vi "ReadMbDat.vi"(0 "ModbusSp in":refnum<class "ModbusSp.lvclass">, 11 "error in (no error)":errorcluster) -> (4 "ModbusSp out":refnum<class "ModbusSp.lvclass">, 6 "Data Read":T1, 8 "register readed":u16[](array[numeric]), 15 "error out":errorcluster)   [LabVIEW 2019, in "ModbusSp.lvclass"]
uses:
  ModbusSp.lvclass
  ReadData.ctl
  ModbusSp.lvclass/ModbusSp.ctl
  Modbus Data Type Conversation/U16 Array TO SGL Array.vi
  <vilib>/NI/Modbus Library/API/Slave/Modbus Slave.lvclass
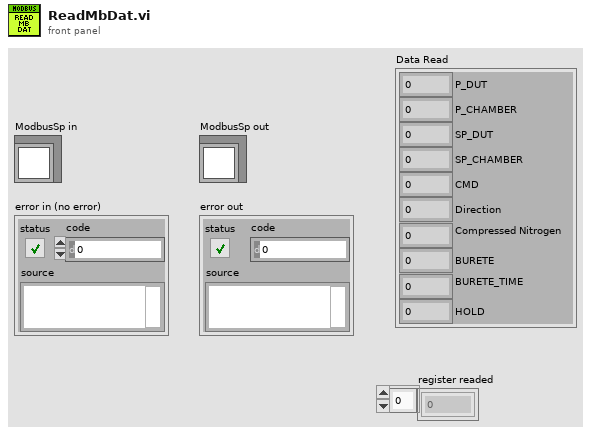
[diagram p1: front panel]
types:
  T1 = typedef "ModbusSp.lvclass/ReadData.ctl" = cluster{"P_DUT":sgl, "P_CHAMBER":sgl, "SP_DUT":sgl, "SP_CHAMBER":sgl, "CMD":u16, "Direction":u16, "Compressed Nitrogen":u16, "BURETE":u16, "BURETE_TIME":u16, "HOLD":u16}
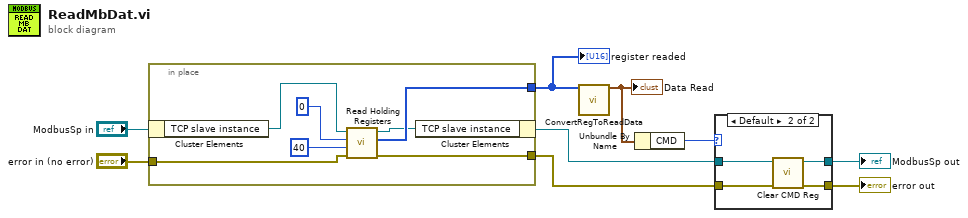
[diagram p0: block diagram]
diagram:
  n1 = in-place {
    in-place-border: "error in (no error)" -> [w15]
    in-place-border: [w12] -> w7
    in-place-border: [w11] -> w3
    n2 = in-place-cluster #1("ModbusSp in") -> ("TCP slave instance"=w16:refnum<class "Modbus Slave.lvclass">)
    n3 = call-dynamic "Read Holding Registers.vi"("error in"=w15, "number of inputs"=u16 40, "starting address"=u16 0, "Modbus slave in"=w16) -> ("error out"=w11:errorcluster, "register values"=w12:u16[], "Modbus slave out"=w10:refnum<class "Modbus Slave.lvclass">)  [unwired: 5 in]
    n4 = in-place-cluster #1("TCP slave instance"=w10) -> (w6:refnum<class "ModbusSp.lvclass">)
  }
  "register readed" <- w7
  n5 = call "ConvertRegToReadData.vi"("register values 0-20"=w7) -> ("data value"=w2:T1)  [unwired: 14 in]
  "Data Read" <- w2
  n6 = Unbundle By Name(w2) -> ("CMD"=w1:u16)
  n7 = case shown="Default" w1 {
    tunnel: w6 -> [w17 w22]
    tunnel: [w18 w21] -> w5
    tunnel: [w17 w20] -> w4
    tunnel: w3 -> [w18 w19]
    frame 0 {
    }
    frame Default {
      n8 = call "Clear CMD Reg.vi"("error in (no error)"=w19, "ModbusSp in"=w22) -> ("error out"=w21:errorcluster, "ModbusSp out"=w20:refnum<class "ModbusSp.lvclass">)  [unwired: 8 in]
    }
  }
  "error out" <- w5
  "ModbusSp out" <- w4
